vi "Temperature with structure case.vi"() -> ()   [LabVIEW 2020]
panel:
  in  "stop":bool
  out "Waveform Chart":dbl(graph)
  in  "F          C":bool
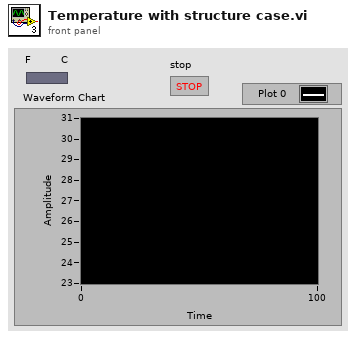
[diagram p1: front panel]
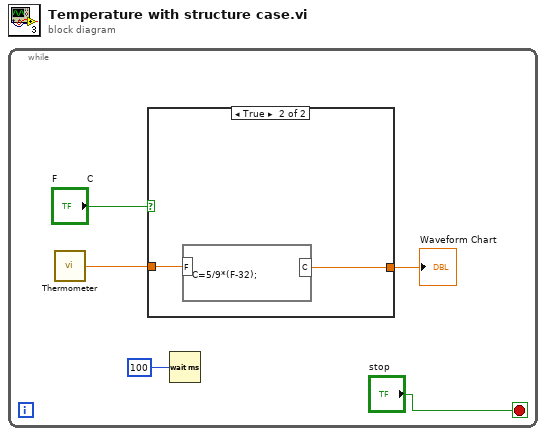
[diagram p0: block diagram]
diagram:
  n1 = while {
    stop <- "stop" stop-if-true
    n2 = call "Thermometer.vi"() -> ("Temperature (deg F)"=w4:dbl)  [unwired: 1 in]
    n3 = case shown="True" "F          C" {
      tunnel: w4 -> [w6 w8]
      tunnel: [w6 w7] -> w3
      frame False {
      }
      frame True {
        n4 = formula code="C=5/9*(F-32);"("F"=w8) -> ("C"=w7:dbl)
      }
    }
    "Waveform Chart" <- w3
    n5 = Wait (ms)(milliseconds to wait=u32 100 ("millisecond timer value")) -> ()  [unwired: 1 out]
  }
